vi "code_infomation.vi"(9 "code":enum16{"无编码", "RS码", "卷积码"}(ring), 10 "signal_in":i8[](array[numeric])) -> (1 "signal_out_for_calclulate_ber":i8[](array[numeric]), 2 "signal_out_code":i8[](array[numeric]))   [LabVIEW 2010]
uses:
  <vilib>/addons/Modulation/Digital/Channel Coding/MT RS Symbol Encoder (shortened).vi
  <vilib>/addons/Modulation/Digital/Channel Coding/MT Convolutional Encoder (Rate).vi
  <vilib>/addons/Modulation/niDMT.lvlib
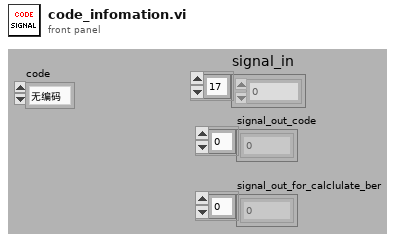
[diagram p1: front panel]
types:
  T1 = typedef "niDMT.lvlib/MT Generic Refnum.ctl" = refnum<k20>
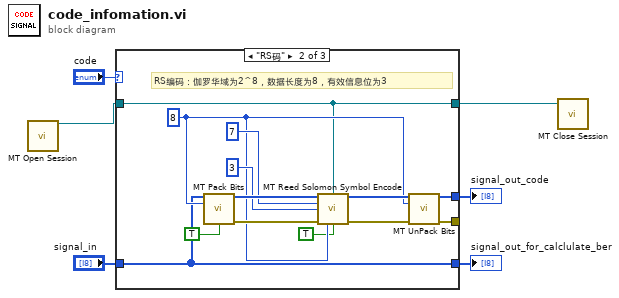
[diagram p0: block diagram]
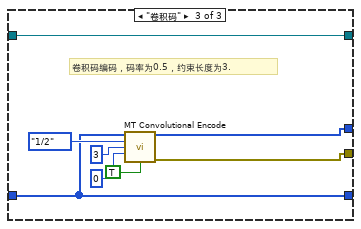
[diagram p3: hidden frame]
diagram:
  n1 = call <vilib>:"MT Open Session.vi"() -> ("modulation session"=w2:T1)  [unwired: 14 in, 1 out]
  n2 = case shown="\"RS码\"" "code" {
    tunnel: [_ w13 w26] -> _
    tunnel: [w8 w14 w25] -> w4
    tunnel: [w8 w12 w24] -> w3
    tunnel: "signal_in" -> [w8 w12 w24]
    tunnel: w2 -> [w7 w10 w23]
    tunnel: [w7 w10 w23] -> w1
    frame "无编码", Default {
    }
    frame "RS码" {
      w15 = 8 ("bits per RS symbol")
      # "RS编码：伽罗华域为2^8，数据长度为8，有效信息位为3"
      n3 = call <vilib>:"MT Pack Bits.vi"("input bit stream"=w12, "bits per integer"=w15, "reset ? (T)"=TRUE) -> ("output integers"=w21:i32[], "error out"=w19:errorcluster)  [unwired: 3 in, 8 out]
      n4 = call-poly <vilib>:"MT Reed Solomon Symbol Encode.vi"("input symbols"=w21, "modulation session"=w10, "code word length (n), symbols"=7, "data word length (k), symbols"=3, "error in (no error)"=w19, "bits per RS symbol"=w15, "reset? (T)"=TRUE) -> ("output symbols"=w20:i32[], "error out"=w18:errorcluster)  [unwired: 7 in]
      n5 = call <vilib>:"MT UnPack Bits.vi"("input integers"=w20, "bits per integer"=w15, "error in (no error)"=w18) -> ("output bit stream"=w14:i8[], "error out"=w13:errorcluster)  [unwired: 2 in, 9 out]
    }
    frame "卷积码" {
      # "卷积码编码，码率为0.5，约束长度为3."
      n6 = call-poly <vilib>:"MT Convolutional Encode.vi"("input bit stream"=w24, "rate (k/n)"=enum16{"1/2", "1/3", "1/4", "2/3", "3/4"}."1/2", "constraint length (K)"=3, "initial state"=u32 0, "reset? (T)"=TRUE) -> ("output bit stream"=w25:i8[], "error out"=w26:errorcluster)  [unwired: 8 in, 1 out]
    }
  }
  "signal_out_code" <- w4
  "signal_out_for_calclulate_ber" <- w3
  n7 = call <vilib>:"MT Close Session.vi"("modulation session"=w1) -> ()  [unwired: 14 in, 1 out]
